vi "AM Demo.vi"() -> ()   [LabVIEW 2020]
uses:
  <vilib>/measure/NI_MABase.lvlib
panel:
  out "Signal + DC Spectrum":cluster{"f0":dbl, "df":dbl, "magnitude":dbl[]}[](graph)
  out "Carrier Spectrum":cluster{"f0":dbl, "df":dbl, "magnitude":dbl[]}[](graph)
  out "Spectrum":cluster{"f0":dbl, "df":dbl, "magnitude":dbl[]}[](graph)
  in  "Signal Frequency":dbl=20.0
  in  "Carrier Frequency":dbl=200.0 step=10.0
  in  "Modulation":dbl=0.7 min=-2.0 step=0.1
  in  "Stop Button":bool
  out "Modulated Signal":waveform(dbl)(graph)={"t0"=timestamp(147.6 s since 1904-01-01), "dt"=0.0001, "Y"=array[3000 elements]}
  out "Signal and DC":waveform(dbl)[](graph)
  out "Carrier Wave":waveform(dbl)(graph)={"t0"=timestamp(147.6 s since 1904-01-01), "dt"=0.0001, "Y"=array[3000 elements]}
  # "Amplitude Modulation"
  # "McClellan et al., DSP First, Example 3-5"
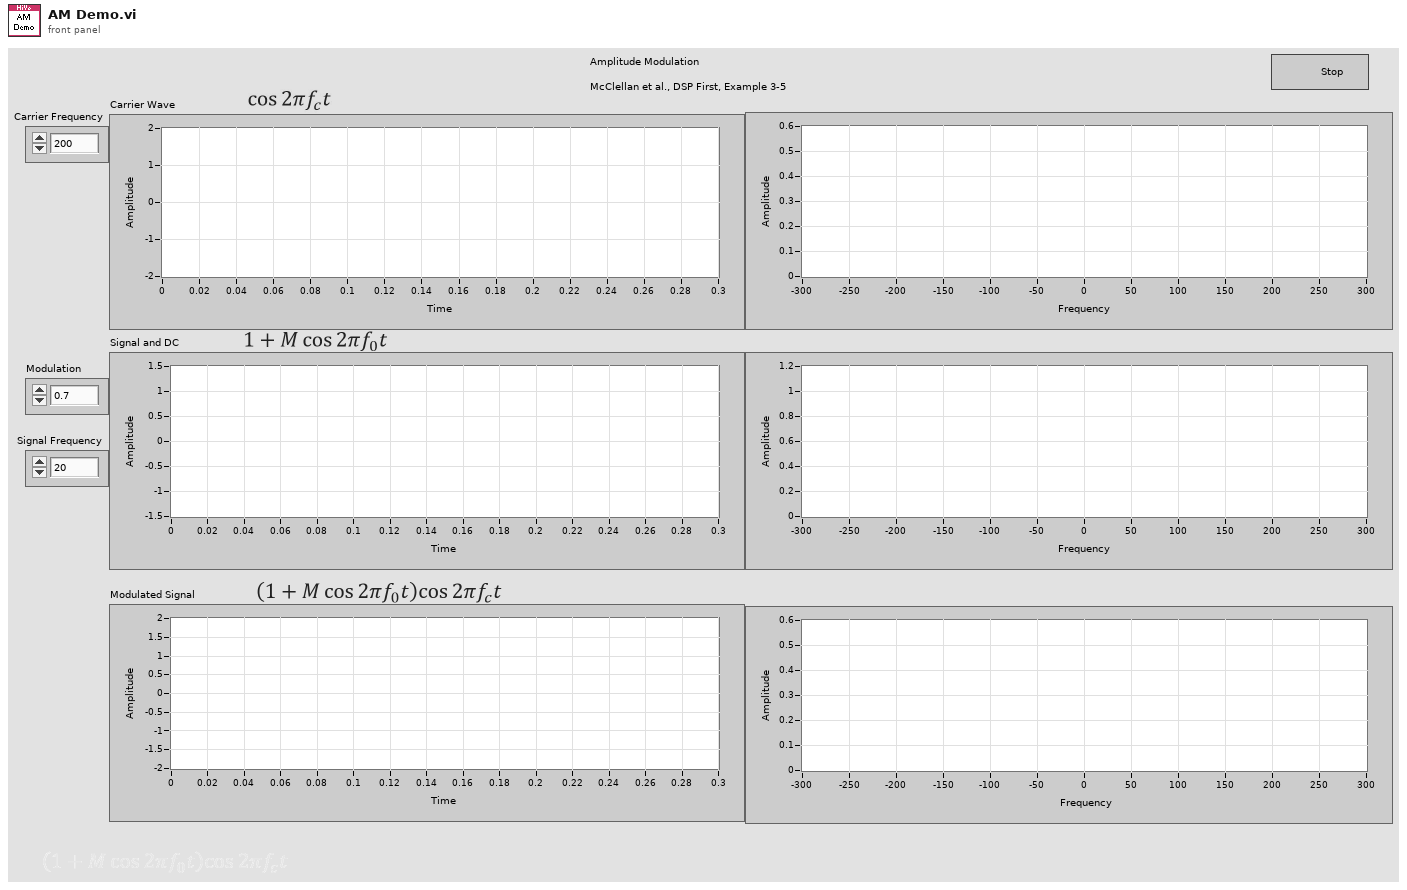
[diagram p1: front panel]
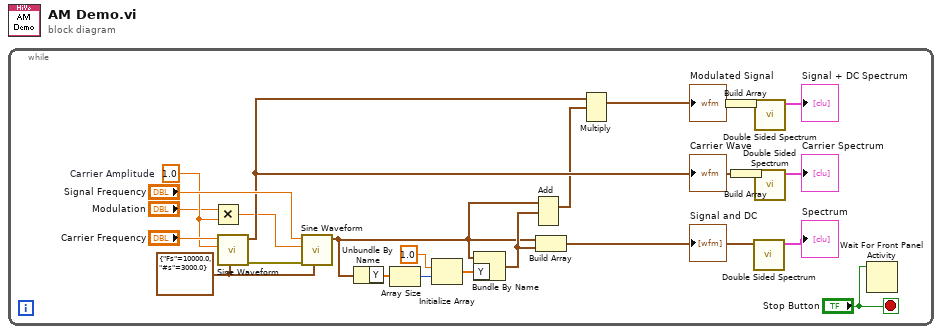
[diagram p0: block diagram]
diagram:
  n1 = while {
    stop <- "Stop Button" stop-if-true
    w13 = 1.0  # Carrier Amplitude
    w20 = cluster{"Fs":dbl, "#s":dbl} {"Fs"=10000.0, "#s"=3000.0} ("sampling info")
    n2 = Multiply(x="Modulation", y=w13) -> (x*y=w11:dbl)
    n3 = call <vilib>:"Sine Waveform.vi"("sampling info"=w20, "amplitude"=w13, "frequency"="Carrier Frequency") -> ("error out"=w21:errorcluster, "signal out"=w18:waveform(dbl))  [unwired: 7 in]
    "Carrier Wave" <- w18
    n4 = call <vilib>:"Sine Waveform.vi"("sampling info"=w20, "error in (no error)"=w21, "amplitude"=w11, "frequency"="Signal Frequency") -> ("signal out"=w4:waveform(dbl))  [unwired: 6 in, 1 out]
    n5 = Unbundle By Name(w4) -> ("Y"=w9:dbl[])
    n6 = Array Size(array=w9) -> (size(s)=w7:i32)
    n7 = Initialize Array(1.0 ("y"), w7) -> (w8:dbl[])
    n8 = Bundle By Name(cluster=w4, "Y"=w8) -> (w5:waveform(dbl))
    n9 = Add(1:w5, 2:w4) -> (0:w10:waveform(dbl))  [unwired: 1 in, 1 out]
    n10 = Build Array(w4, w5) -> (w3:waveform(dbl)[])
    "Signal and DC" <- w3
    n11 = Multiply(1:w10, 2:w18) -> (0:w15:waveform(dbl))  [unwired: 1 in, 1 out]
    "Modulated Signal" <- w15
    n12 = Build Array(w15) -> (w1:waveform(dbl)[])
    n13 = Build Array(w18) -> (w2:waveform(dbl)[])
    n14 = call "Double Sided Spectrum.vi"("Signals In"=w3) -> ("Double Sided Spectra"=→"Spectrum":cluster{"f0":dbl, "df":dbl, "magnitude":dbl[]}[])  [unwired: 9 in, 1 out]
    n15 = call "Double Sided Spectrum.vi"("Signals In"=w1) -> ("Double Sided Spectra"=→"Signal + DC Spectrum":cluster{"f0":dbl, "df":dbl, "magnitude":dbl[]}[])  [unwired: 9 in, 1 out]
    n16 = call "Double Sided Spectrum.vi"("Signals In"=w2) -> ("Double Sided Spectra"=→"Carrier Spectrum":cluster{"f0":dbl, "df":dbl, "magnitude":dbl[]}[])  [unwired: 9 in, 1 out]
    n17 = Wait For Front Panel Activity(3:"Stop Button") -> ()  [unwired: 2 in, 1 out]
  }
